vi "LoopVI-V6.vi"() -> ()   [LabVIEW 2013]
uses:
  <vilib>/Utility/file.llb/Read From Spreadsheet File (DBL).vi
panel:
  out "min index(es)":i32
  out "min value":dbl
  out "output array":dbl[](array[numeric])
  out "Collimator afstand":dbl
  out "Spleedbreedte":dbl
  out "Alignment correction":dbl
  out "Background coincidence counts":dbl
  out "Core width":dbl
  out "Fermi Angle":dbl
  out "22na source radius":dbl
  out "Fraction core annihilations":dbl
  out "Minimum summed squared residuals":dbl
  in  "Step size":dbl=1.0 format="%#_13g"
  in  "Begin range":dbl=575.0 format="%#_13g"
  in  "Amount of steps":i32=50
  in  "?":dbl=0.1 format="%#_13g"
  in  "Begin range":dbl=0.5 format="%#_13g"
  in  "Amount of steps":i32=10
  in  "Step size":dbl=0.1 format="%#_13g"
  in  "Begin range":dbl=2.5 format="%#_13g"
  in  "Amount of steps":i32=40
  in  "Step size":dbl=0.1 format="%#_13g"
  in  "Begin range":dbl=1.0 format="%#_13g"
  in  "Amount of steps":dbl=10.0 format="%#_13g"
  in  "Step size":dbl=0.1 format="%#_13g"
  in  "Begin range":dbl=4.0 format="%#_13g"
  in  "Amount of steps":i32=5
  in  "Amount of steps":dbl=4.0 format="%#_13g"
  in  "Step size":dbl=0.1 format="%#_13g"
  in  "Amount of steps":i32=20
  in  "Amount of steps":i32=2
  in  "Begin range":dbl=6.5 format="%#_13g"
  in  "Step size":dbl=0.1 format="%#_13g"
  in  "Begin range":dbl=0.01 format="%#_13g"
  in  "Step size":dbl=0.1 format="%#_13g"
  in  "Begin range":dbl=0.15 format="%#_13g"
  in  "Stop Button":bool
  out "Percentage":dbl format="%#_4f"
  in  "file path (dialog if empty)":path
  in  "Load":bool caption="measurement file\n\n         ??. txt"
  out "free gas model":cluster{"Y":dbl[], "Y":dbl[]}[](graph)
  out "Fermi angle\n   (mrad)":dbl=7.0
  in  "stop 2":bool
  out "core electrons":cluster{"Y":dbl[], "Y":dbl[]}[](graph)
  out "core width\n   (mrad)":dbl=5.0
  out "fraction core\nannihilations":dbl=0.2 min=0.0 max=1.0 step=1e-05
  out "ZICHT  functie":cluster{"Y":dbl[], "Y":dbl[]}[](graph)
  out "spleetbreedte\n      (mm)":dbl=1.0 min=0.1 max=5.0
  out "collimator afstand\n       (mm)":dbl=500.0 min=100.0 max=1000.0
  in  "stop 4":bool
  out "XY Graph 4":cluster{ext[], "Array out":ext[]}[](graph)
  out "alignment correction":dbl min=-10.0 max=10.0 step=0.0001
  out "background \n coincidence counts":dbl min=0.0 max=100.0
  out "Fermi energy (eV)":dbl format="%#_3g"
  out "22Na source radius (mm)":dbl=0.1 min=1e-05 max=3.0
  in  "1d - Acar":bool caption="2d - Acar or DB"
  out "2d - Acar 2":bool
  out "2d - Acar 3":bool
  out "2d - Acar 4":bool
  out "XY Graph 5":cluster{ext[], "Array out":ext[]}[](graph)
  out "output cluster 2":cluster{ext[], ext[]}
  out "Sum of squared residuals":dbl
  in  "sigma (mrad) 2":dbl
  # "Step size"
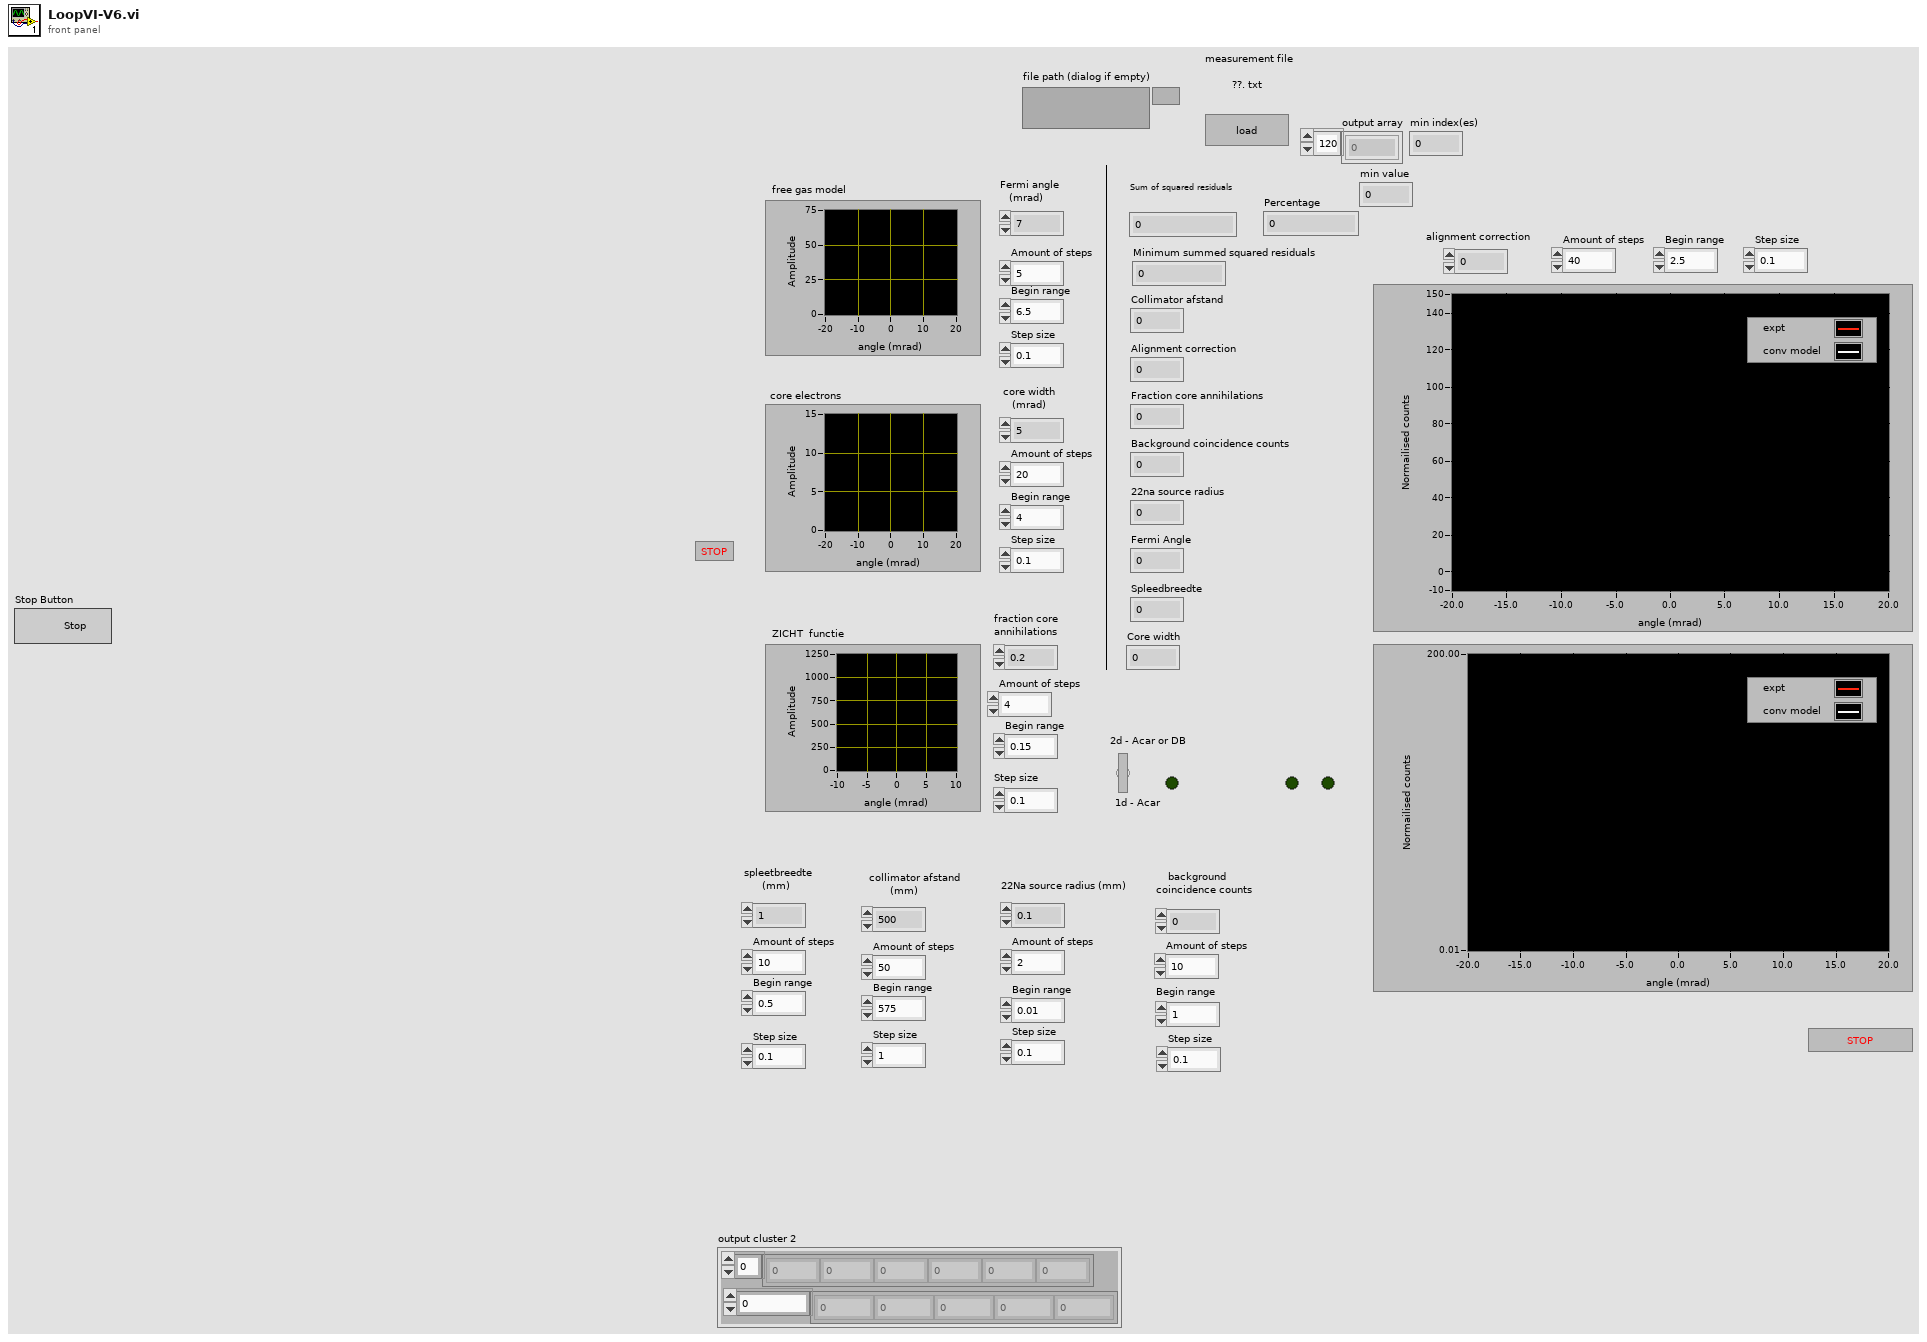
[diagram p1: front panel]
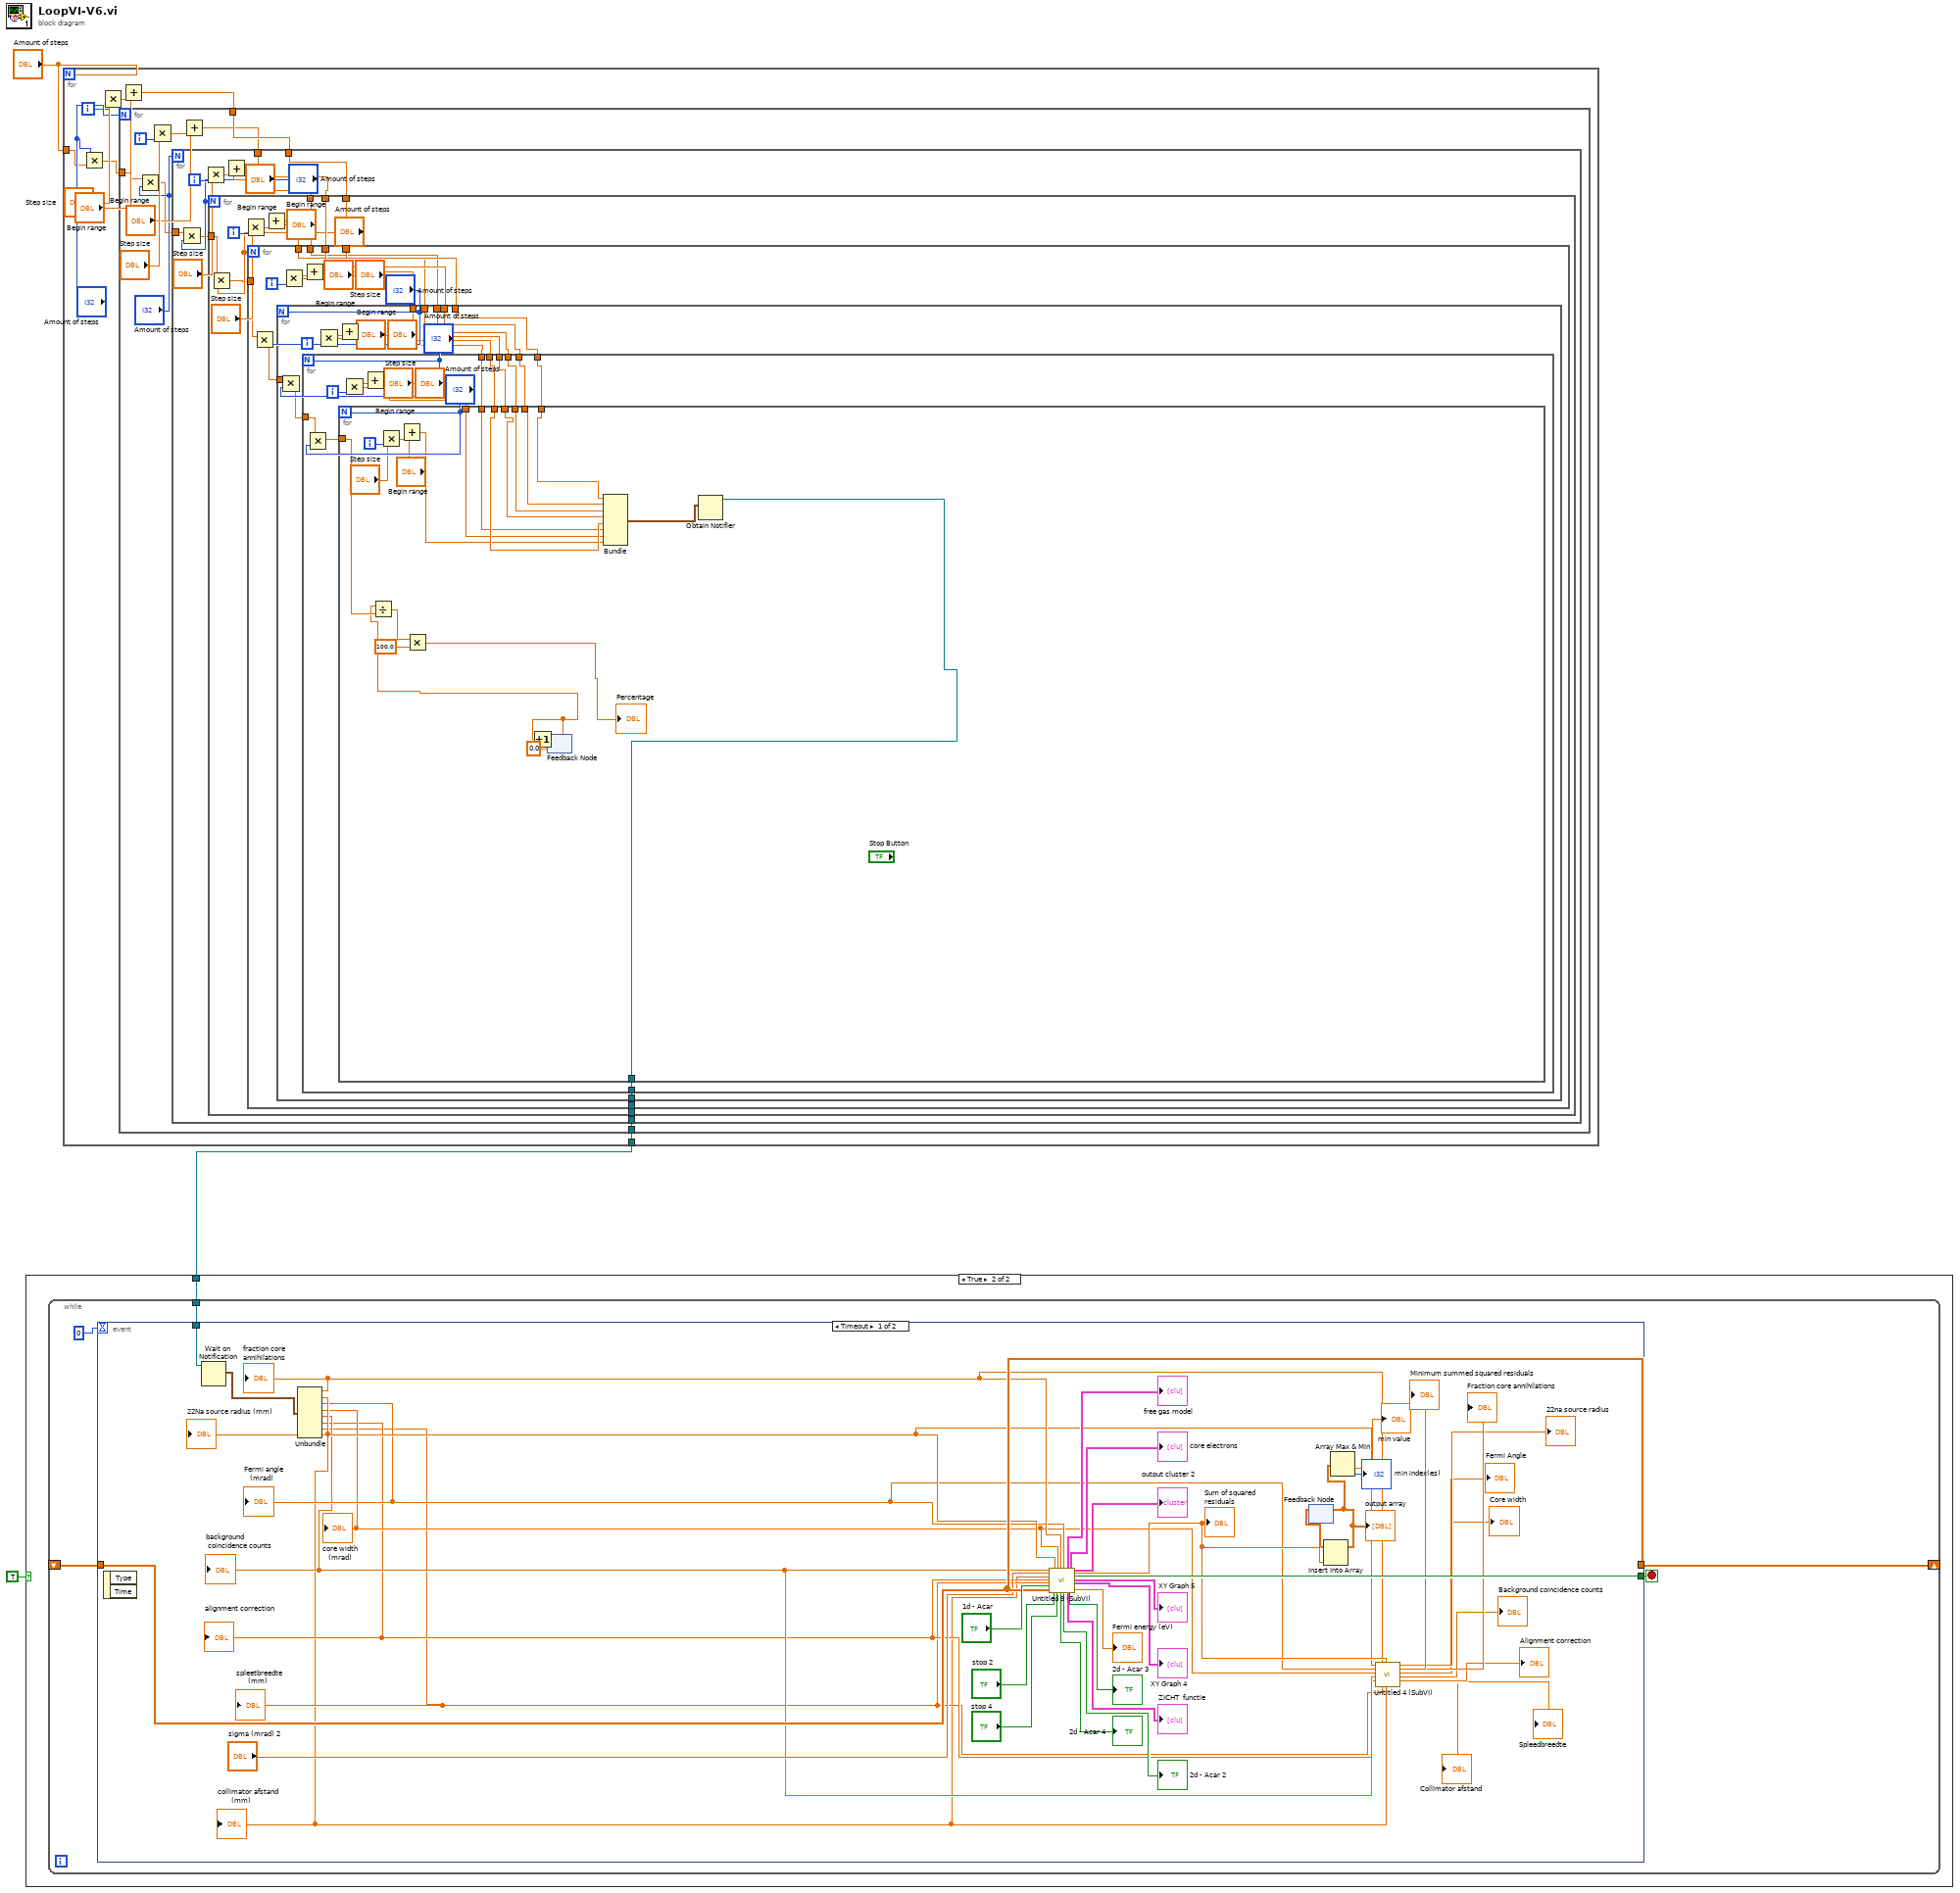
[diagram p0: block diagram]
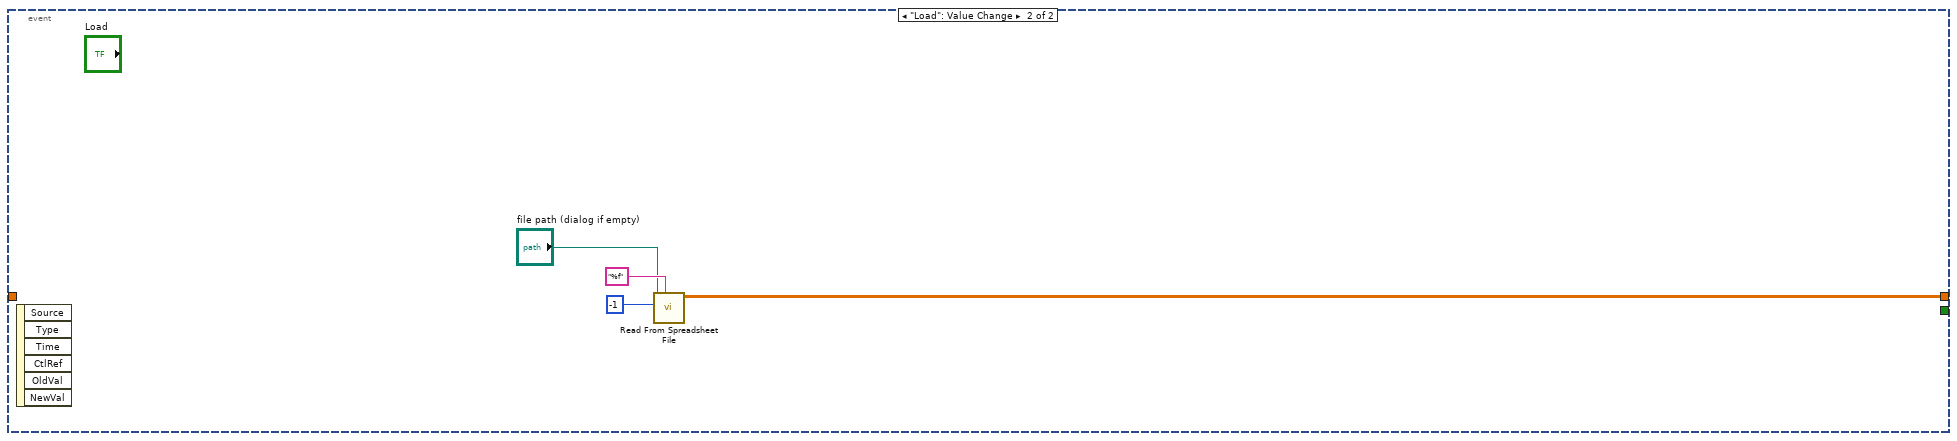
[diagram p3: hidden frame]
diagram:
  n1 = for {
    N: "Amount of steps" -> [_]
    tunnel: "Amount of steps" -> [w7]
    tunnel: [w4] -> w1
    i -> [w5]
    n2 = Multiply(x="Amount of steps", y=w7) -> (x*y=w6:dbl)
    n3 = Multiply(x="Step size", y=w5) -> (x*y=w11:dbl)
    n4 = Add(x="Begin range", y=w11) -> (x+y=w9:dbl)
    n5 = for {
      N: "Amount of steps" -> [_]
      tunnel: w9 -> [w18]
      tunnel: w6 -> [w16]
      tunnel: [w13] -> w4
      i -> [w22]
      n6 = Multiply(x=w16, y="Amount of steps") -> (x*y=w14:dbl)
      n7 = Multiply(x="Step size", y=w22) -> (x*y=w20:dbl)
      n8 = Add(x="Begin range", y=w20) -> (x+y=w17:dbl)
      n9 = for {
        N: "Amount of steps" -> [_]
        tunnel: w18 -> [w29]
        tunnel: w17 -> [w28]
        tunnel: w14 -> [w26]
        tunnel: [w23] -> w13
        i -> [w33]
        n10 = Multiply(x=w26, y="Amount of steps") -> (x*y=w24:dbl)
        n11 = Multiply(x="Step size", y=w33) -> (x*y=w31:dbl)
        n12 = Add(x="Begin range", y=w31) -> (x+y=w27:dbl)
        n13 = for {
          N: "Amount of steps" -> [_]
          tunnel: w29 -> [w38]
          tunnel: w28 -> [w39]
          tunnel: w27 -> [w40]
          tunnel: w24 -> [w37]
          tunnel: [w34] -> w23
          i -> [w45]
          n14 = Multiply(x=w37, y="Amount of steps") -> (x*y=w35:dbl)
          n15 = Multiply(x="Step size", y=w45) -> (x*y=w43:dbl)
          n16 = Add(x="Begin range", y=w43) -> (x+y=w41:dbl)
          n17 = for {
            N: "Amount of steps" -> [_]
            tunnel: w41 -> [w51]
            tunnel: w40 -> [w52]
            tunnel: w39 -> [w53]
            tunnel: w38 -> [w54]
            tunnel: w35 -> [w49]
            tunnel: [w46] -> w34
            i -> [w58]
            n18 = Multiply(x=w49, y="Amount of steps") -> (x*y=w47:dbl)
            n19 = Multiply(x="Step size", y=w58) -> (x*y=w56:dbl)
            n20 = Add(x="Begin range", y=w56) -> (x+y=w50:dbl)
            n21 = for {
              N: "Amount of steps" -> [_]
              tunnel: w54 -> [w68]
              tunnel: w53 -> [w67]
              tunnel: w52 -> [w66]
              tunnel: w51 -> [w65]
              tunnel: w50 -> [w64]
              tunnel: w47 -> [w62]
              tunnel: [w59] -> w46
              i -> [w72]
              n22 = Multiply(x=w62, y="Amount of steps") -> (x*y=w60:dbl)
              n23 = Multiply(x="Step size", y=w72) -> (x*y=w70:dbl)
              n24 = Add(x="Begin range", y=w70) -> (x+y=w63:dbl)
              n25 = for {
                N: "Amount of steps" -> [_]
                tunnel: w68 -> [w82]
                tunnel: w67 -> [w81]
                tunnel: w66 -> [w80]
                tunnel: w65 -> [w79]
                tunnel: w64 -> [w78]
                tunnel: w63 -> [w77]
                tunnel: w60 -> [w76]
                tunnel: [w73] -> w59
                i -> [w87]
                n26 = Multiply(x=w76, y="Amount of steps") -> (x*y=w74:dbl)
                n27 = Multiply(x="?", y=w87) -> (x*y=w85:dbl)
                n28 = Add(x="Begin range", y=w85) -> (x+y=w83:dbl)
                n29 = for {
                  N: "Amount of steps" -> [_]
                  tunnel: w83 -> [w91]
                  tunnel: w82 -> [w97]
                  tunnel: w81 -> [w96]
                  tunnel: w80 -> [w95]
                  tunnel: w79 -> [w94]
                  tunnel: w78 -> [w93]
                  tunnel: w77 -> [w92]
                  tunnel: w74 -> [w102]
                  tunnel: [w88] -> w73
                  i -> [w108]
                  n30 = Multiply(x="Step size", y=w108) -> (x*y=w106:dbl)
                  n31 = Add(x="Begin range", y=w106) -> (x+y=w90:dbl)
                  n32 = feedback #1(0.0) -> (w101:dbl)
                  n33 = Divide(x=w101, y=w102) -> (x/y=w100:dbl)
                  n34 = Multiply(x=w100, y=100.0) -> (x*y=→"Percentage":dbl)
                  n35 = Increment(x=w101) -> (x+1=w104:dbl)
                  n36 = feedback-in #1(w104) -> ()
                  n37 = Bundle(w97, w96, w95, w94, w93, w92, w91, w90) -> (w89:cluster{dbl, dbl, dbl, dbl, dbl, dbl, dbl, dbl})  [unwired: 1 in]
                  n38 = Obtain Notifier(notification data type=w89) -> (notifier out=w88:refnum<notifier>)  [unwired: 3 in, 2 out]
                }
              }
            }
          }
        }
      }
    }
  }
  n39 = case shown="True" TRUE {
    tunnel: w1 -> [_ w109]
    frame False {
    }
    frame True {
      n40 = while {
        shift-right: [w112] -> _
        shift-left: _ -> [w111]
        tunnel: w109 -> [w110]
        stop <- w114 stop-if-true
        n41 = event shown="[0] Timeout" {
          selector: _ -> [_ _]
          dyn-events: _ -> [_ _]
          timeout: 0 -> [_ _]
          tunnel: [w154 _] -> w114
          tunnel: [w152 w157] -> w112
          tunnel: w111 -> [w152 _]
          tunnel: w110 -> [w124 _]
          event Timeout {
            n42 = event-data() -> ()  [unwired: 1 in, 2 out]
            n43 = Wait on Notification(notifier=w124) -> (notification=w123:cluster{dbl, dbl, dbl, dbl, dbl, dbl, dbl, dbl})  [unwired: 3 in, 3 out]
            n44 = Unbundle(w123) -> (w122:dbl, w121:dbl, w120:dbl, w119:dbl, w118:dbl, w117:dbl, w116:dbl, w115:dbl)
            "Fermi angle\n   (mrad)" <- w120
            "core width\n   (mrad)" <- w119
            "fraction core\nannihilations" <- w122
            "spleetbreedte\n      (mm)" <- w116
            "collimator afstand\n       (mm)" <- w115
            "alignment correction" <- w117
            "background \n coincidence counts" <- w118
            "22Na source radius (mm)" <- w121
            n45 = call "Untitled 9 (SubVI).vi"("background \n coincidence counts"=w118, "sigma (mrad) in"="sigma (mrad) 2", "collimator afstand\n       (mm)"=w115, "alignment correction"=w117, "spleetbreedte\n      (mm)"=w116, "1d - Acar"="1d - Acar", "all rows"=w152, "22Na source radius (mm)"=w121, "stop in"="stop 2", "core width\n   (mrad)"=w119, "stop 4"="stop 4", "fraction core\nannihilations"=w122, "Fermi angle\n   (mrad)"=w120) -> ("2d - Acar 4"=→"2d - Acar 4":bool, "2d - Acar 2"=→"2d - Acar 2":bool, "free gas model"=→"free gas model":cluster{"Y":dbl[], "Y":dbl[]}[], "ZICHT  functie"=→"ZICHT  functie":cluster{"Y":dbl[], "Y":dbl[]}[], "core electrons"=→"core electrons":cluster{"Y":dbl[], "Y":dbl[]}[], "2d - Acar 3"=→"2d - Acar 3":bool, "output cluster 2"=→"output cluster 2":cluster{ext[], ext[]}, "Sum of squared residuals"=w129:dbl, "stop 3"=w154:bool, "XY Graph 5"=→"XY Graph 5":cluster{ext[], "Array out":ext[]}[], "XY Graph 4"=→"XY Graph 4":cluster{ext[], "Array out":ext[]}[], "Fermi energy (eV)"=→"Fermi energy (eV)":dbl)  [unwired: 2 in, 1 out]
            "Sum of squared residuals" <- w129
            n46 = feedback #2() -> (w128:dbl[])  [unwired: 1 in]
            n47 = Insert Into Array(array=w128, new element=w129) -> (w127:dbl[])  [unwired: 1 in]
            "output array" <- w127
            n48 = feedback-in #2(w127) -> ()
            n49 = Array Max & Min(array=w127) -> (min value=→"min value":dbl, min index (indices)=→"min index(es)":i32)  [unwired: 2 out]
            n50 = call "Untitled 4 (SubVI).vi"("x 19"=w121, "x 18"=w120, "x 17"=w119, "x 16"=w118, "x 15"=w117, "x 20"=w122, "x 14"=w116, "x 4"=w129, "x 13"=w115) -> ("x 3"=→"Minimum summed squared residuals":dbl, "x 12"=→"Collimator afstand":dbl, "x 5"=→"Fraction core annihilations":dbl, "x 11"=→"Spleedbreedte":dbl, "x 6"=→"22na source radius":dbl, "x 7"=→"Fermi Angle":dbl, "x 8"=→"Core width":dbl, "x 9"=→"Background coincidence counts":dbl, "x 10"=→"Alignment correction":dbl)  [unwired: 2 in]
          }
          event "Load": Value Change {
            n51 = event-data() -> ()  [unwired: 1 in, 6 out]
            n52 = call-poly <vilib>:"Read From Spreadsheet File.vi"("format (%.3f)"="%f", "number of rows (all:-1)"=-1, "file path (dialog if empty)"="file path (dialog if empty)") -> ("all rows"=w157:ext[][])  [unwired: 4 in, 4 out]
          }
        }
      }
    }
  }
